vi "CLOSE_HSDIO.vi"(8 "Error In":errorcluster, 11 "HSDIO Sessions":T1) -> (0 "Error Out":errorcluster)   [LabVIEW 2013]
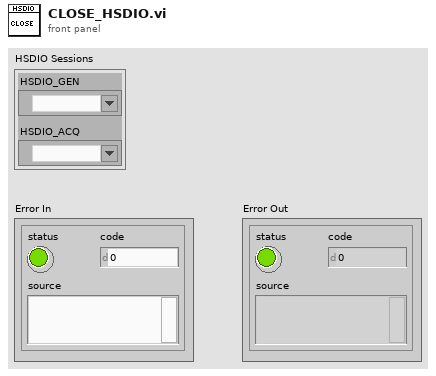
[diagram p1: front panel]
types:
  T1 = cluster{"HSDIO_ACQ":refnum<k15>, "HSDIO_GEN":refnum<k15>}
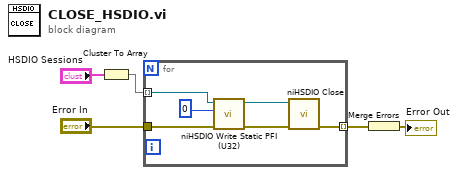
[diagram p0: block diagram]
diagram:
  n1 = Cluster To Array(cluster="HSDIO Sessions") -> (array=w4:refnum<k15>[])
  n2 = for {
    tunnel: w4 -> [w6] mode=indexing
    tunnel: "Error In" -> [w10]
    tunnel: [w11] -> w2 mode=indexing
    n3 = call <instrlib>:"niHSDIO Write Static PFI (U32).vi"("error in (no error)"=w10, "write data (0x0000)"=u32 0, "instrument handle"=w6) -> ("error out"=w9:errorcluster, "instrument handle out"=w8:refnum<k15>)  [unwired: 7 in]
    n4 = call <instrlib>:"niHSDIO Close.vi"("error in (no error)"=w9, "instrument handle"=w8) -> ("error out"=w11:errorcluster)  [unwired: 9 in]
  }
  n5 = Merge Errors(w2) -> (→"Error Out":errorcluster)
